vi "AdaptToInputs.vi"(3 "Term Types":T1, 4 "XRef":refnum<vi>, 5 "State In":T5) -> (0 "Reply":string[](array[string]), 2 "State Out":T5)   [LabVIEW 2018, in "OpenG Slice 1D Array.xnode"]
uses:
  OpenG Slice 1D Array.xnode
  State.ctl
  <vilib>/XNodeSupport/XNodeTermTypeIDPairs.ctl
  <vilib>/XNodeSupport/XNodeTermTypeIDPair.ctl
  <vilib>/XNodeSupport/XNodeType.ctl
  <vilib>/XNodeSupport/XNodeString.ctl
  <userlib>/_LAVAcr/Scripting Tools/XNode Support/TypeDefs/Array Dimension Tests.ctl
  <userlib>/_LAVAcr/Scripting Tools/XNode Support/Find term type by ID_type.vi
  <userlib>/_LAVAcr/Scripting Tools/XNode Support/XNode Support.lvlib
  <vilib>/XNodeSupport/NI_XNodeSupport.lvlib
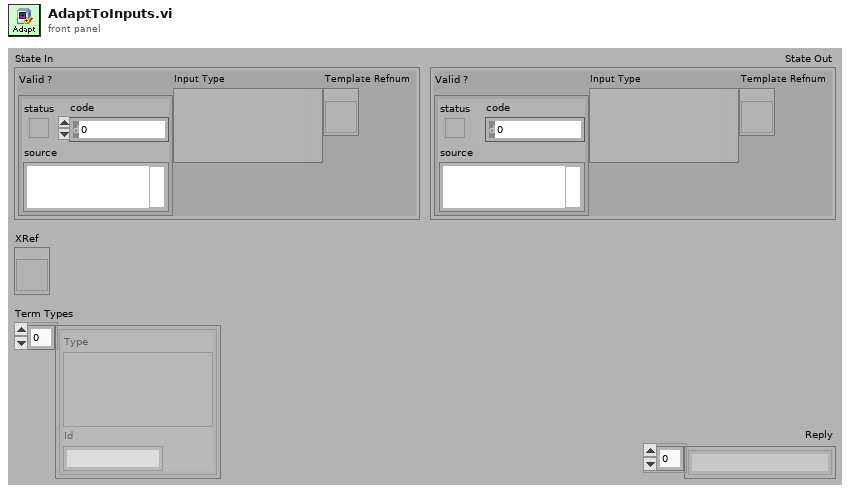
[diagram p1: front panel]
types:
  T1 = typedef "NI_XNodeSupport.lvlib/XNodeTermTypeIDPairs.ctl" = T2[]
  T2 = typedef "NI_XNodeSupport.lvlib/XNodeTermTypeIDPair.ctl" = cluster{"Type":T3, "Id":T4}
  T3 = typedef "NI_XNodeSupport.lvlib/XNodeType.ctl" = variant
  T4 = typedef "NI_XNodeSupport.lvlib/XNodeString.ctl" = string
  T5 = typedef "OpenG Slice 1D Array.xnode/State.ctl" = cluster{"Valid ?":errorcluster, "Input Type":variant, "Template Refnum":refnum<vi>}
  T6 = typedef "Scripting Tools.lvlib/XNode Support.lvlib/Array Dimension Tests.ctl" = enum16{"No Check", "At Least n dimensions", "Exactly N Dimensions", "No More Than N Dimensions"}
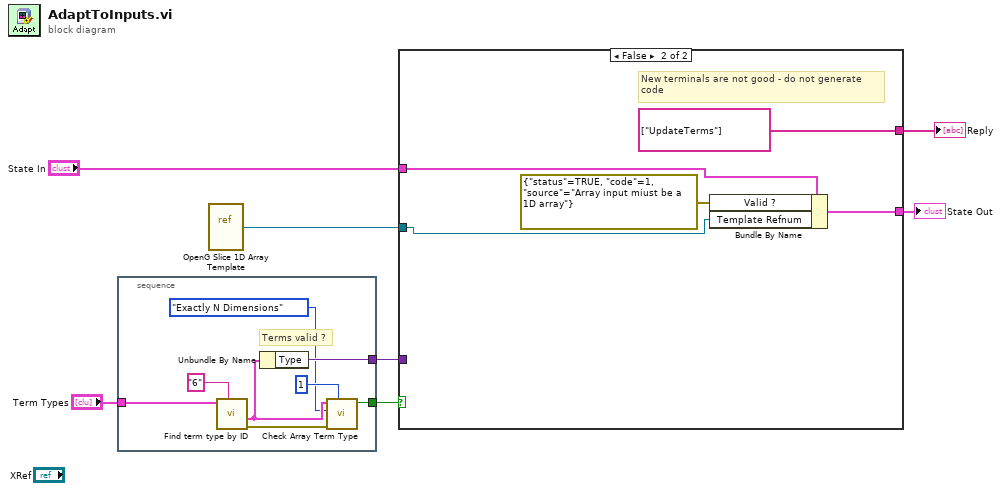
[diagram p0: block diagram]
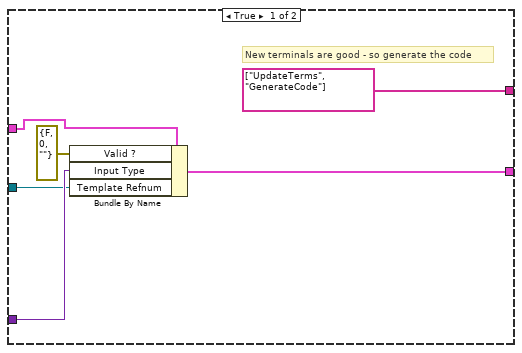
[diagram p2: hidden frame]
diagram:
  n1 = stacked-sequence {
    tunnel: "Term Types" -> [w15]
    tunnel: [w8] -> w6
    tunnel: [w13] -> w2
    frame #0 {
      # "Terms valid ?"
      n2 = call-poly <userlib>:"Find term type by ID.vi"("Search ID"="6", "Term Types"=w15) -> ("error out"=w9:errorcluster, "Term Type"=w12:T2)  [unwired: 1 in, 7 out]
      n3 = Unbundle By Name(w12) -> ("Type"=w13:T3)
      n4 = call <userlib>:"Check Array Term Type.vi"("Dimensions Required"=1, "error in (no error)"=w9, "Dimension Check"=Array_Dimension_Tests."Exactly N Dimensions", "Term Type"=w12) -> ("Is Good ?"=w8:bool)  [unwired: 1 in, 6 out]
    }
  }
  n5 = vi-ref "OpenG Slice 1D Array Template.vi"() -> (w1:refnum<vi>)
  n6 = case shown="False" w6 {
    tunnel: "State In" -> [w21 w26]
    tunnel: [w19 w24] -> w4
    tunnel: [string[] ["UpdateTerms", "GenerateCode"] ("Reply") string[] ["UpdateTerms"] ("Reply")] -> w3
    tunnel: w2 -> [w17 _]
    tunnel: w1 -> [w16 w22]
    frame True {
      # "New terminals are good - so generate the code"
      n7 = Bundle By Name(cluster=w21, "Valid ?"=errorcluster {"status"=FALSE, "code"=0, "source"=""}, "Input Type"=w17, "Template Refnum"=w16) -> (w19:T5)
    }
    frame False {
      # "New terminals are not good - do not generate\ncode"
      n8 = Bundle By Name(cluster=w26, "Valid ?"=errorcluster {"status"=TRUE, "code"=1, "source"="Array input miust be a 1D array"}, "Template Refnum"=w22) -> (w24:T5)
    }
  }
  "Reply" <- w3
  "State Out" <- w4
